vi "writetestreport.vi"(9 "test report":T1(array[cluster])) -> ()   [LabVIEW 2012]
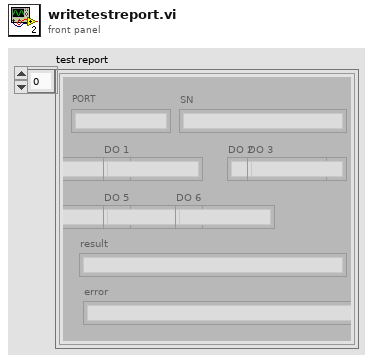
[diagram p1: front panel]
types:
  T1 = cluster{"PORT":string, "SN":string, "DO 0":string, "DO 1":string, "DO 2":string, "DO 3":string, "DO 4":string, "DO 5":string, "DO 6":string, "result":string, "error":string}[]
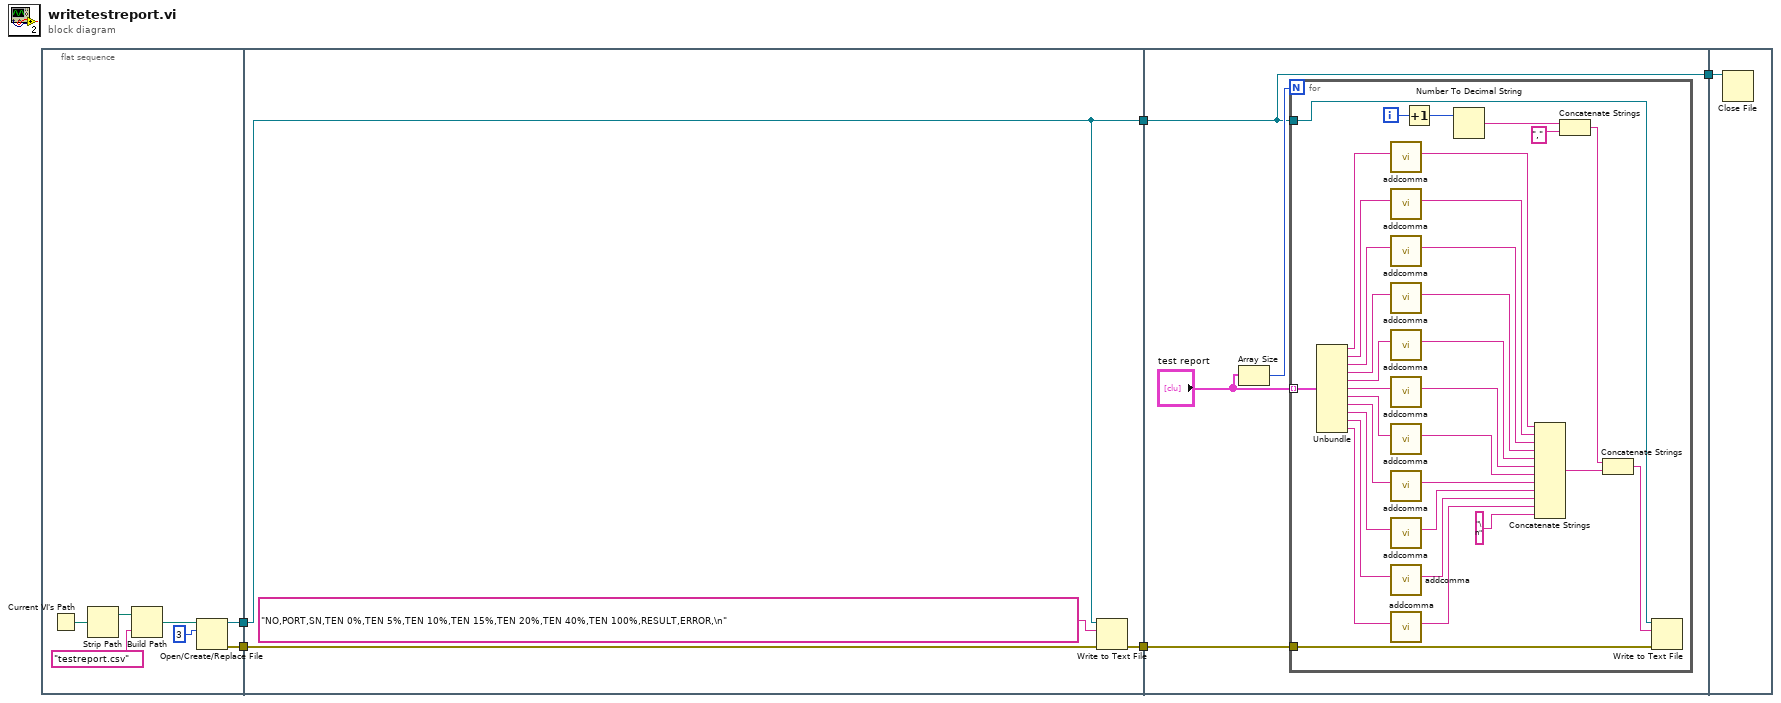
[diagram p0: block diagram]
diagram:
  n1 = flat-sequence {
    tunnel: [w7] -> w5
    tunnel: [w6] -> w4
    tunnel: w5 -> [w14]
    tunnel: w4 -> [w15]
    tunnel: [w14] -> w3
    tunnel: [w13] -> w2
    tunnel: w3 -> [w18]
    tunnel: w2 -> [w19]
    tunnel: [w18] -> w1
    tunnel: w1 -> [w54]
    frame #0 {
      n2 = Current VI's Path() -> (path=w8:path)
      n3 = Strip Path(path=w8) -> (stripped path=w9:path)  [unwired: 1 out]
      n4 = Build Path(base path=w9, name or relative path="testreport.csv") -> (appended path=w12:path)
      n5 = Open/Create/Replace File(file path (use dialog)=w12, operation (0:open)=3) -> (refnum out=w7:refnum<file>, error out=w6:errorcluster)  [unwired: 4 in, 1 out]
    }
    frame #1 {
      n6 = Write to Text File(file (use dialog)=w14, text="NO,PORT,SN,TEN 0%,TEN 5%,TEN 10%,TEN 15%,TEN 20%,TEN 40%,TEN 100%,RESULT,ERROR,\n", error in=w15) -> (error out=w13:errorcluster)  [unwired: 1 in, 2 out]
    }
    frame #2 {
      n7 = Array Size(array="test report") -> (size(s)=w20:i32)
      n8 = for {
        N: w20 -> [_]
        tunnel: "test report" -> [w53] mode=indexing
        tunnel: w18 -> [w48]
        tunnel: w19 -> [w47]
        i -> [w41]
        n9 = Unbundle(w53) -> ("PORT"=w51:string, "SN"=w52:string, "DO 0"=w34:string, "DO 1"=w32:string, "DO 2"=w29:string, "DO 3"=w21:string, "DO 4"=w22:string, "DO 5"=w24:string, "DO 6"=w23:string, "result"=w39:string, "error"=w37:string)
        n10 = call "addcomma.vi"("INPUT"=w51) -> ("OUTPUT"=w50:string)  [unwired: 10 in]
        n11 = call "addcomma.vi"("INPUT"=w52) -> ("OUTPUT"=w49:string)  [unwired: 10 in]
        n12 = call "addcomma.vi"("INPUT"=w34) -> ("OUTPUT"=w33:string)  [unwired: 10 in]
        n13 = call "addcomma.vi"("INPUT"=w32) -> ("OUTPUT"=w31:string)  [unwired: 10 in]
        n14 = call "addcomma.vi"("INPUT"=w29) -> ("OUTPUT"=w30:string)  [unwired: 10 in]
        n15 = call "addcomma.vi"("INPUT"=w21) -> ("OUTPUT"=w28:string)  [unwired: 10 in]
        n16 = call "addcomma.vi"("INPUT"=w22) -> ("OUTPUT"=w27:string)  [unwired: 10 in]
        n17 = call "addcomma.vi"("INPUT"=w24) -> ("OUTPUT"=w25:string)  [unwired: 10 in]
        n18 = call "addcomma.vi"("INPUT"=w23) -> ("OUTPUT"=w26:string)  [unwired: 10 in]
        n19 = call "addcomma.vi"("INPUT"=w39) -> ("OUTPUT"=w38:string)  [unwired: 10 in]
        n20 = call "addcomma.vi"("INPUT"=w37) -> ("OUTPUT"=w36:string)  [unwired: 10 in]
        n21 = Increment(x=w41) -> (x+1=w40:i32)
        n22 = Number To Decimal String(number=w40) -> (decimal integer string=w44:string)  [unwired: 1 in]
        n23 = Concatenate Strings(w50, w49, w33, w31, w30, w28, w27, w25, w26, w38, w36, "\n") -> (w46:string)
        n24 = Concatenate Strings(w44, ",") -> (w42:string)
        n25 = Concatenate Strings(w42, w46) -> (w45:string)
        n26 = Write to Text File(file (use dialog)=w48, text=w45, error in=w47) -> ()  [unwired: 1 in, 3 out]
      }
    }
    frame #3 {
      n27 = Close File(refnum=w54) -> ()  [unwired: 1 in, 2 out]
    }
  }
